vi "create Complex Data.vi"() -> (0 "error out":errorcluster, 1 "Complex Data":refnum<class "Complex Data.lvclass">)   [LabVIEW 2017]
doc: "Creates a Complex Data object."
uses:
  Program Files/Thorlabs/SpectralRadar/LabVIEW/2012/user.lib/SpectralRadar.llb/Complex Data.lvclass
  SpectralRadar.dll
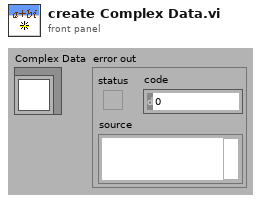
[diagram p1: front panel]
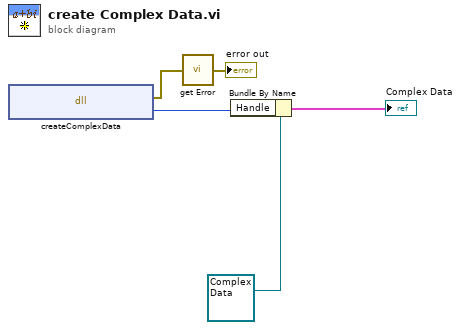
[diagram p0: block diagram]
diagram:
  n1 = dll-call lib="SpectralRadar.dll" fn="createComplexData"() -> (error out=w2:errorcluster, "Complex Data Handle"=w5:u64)  [unwired: 3 in, 1 out]
  n2 = call "get Error.vi"("error in (no error)"=w2) -> ("error out"=→"error out":errorcluster)
  n3 = Bundle By Name(cluster=refnum<class "Complex Data.lvclass"> refnum ("ComplexData.lvclass"), "Handle"=w5) -> (→"Complex Data":cluster{})
